vi "Vision Code.vi"(0 "Image In":T1, 1 "Image Dst":T1, 2 "Final Image Output":T1, 7 "error in":errorcluster) -> (20 "Image Out":T1, 22 "Output Image":T1(plugin-control), 27 "error out":errorcluster)   [LabVIEW 2014]
doc: "Creates, edits, and runs vision algorithms using NI Vision Assistant.\n\nWhen you place this Express VI on the block diagram, NI Vision Assistant launches. Create an algorithm using the Vision Assistant processing functions. After you create an algorithm, you can select the controls and indicators that you want to be able to programmatically set in LabVIEW. Double-click the Vision Assistant Express VI to edit the algorithm."
uses:
  <vilib>/vision/Image Controls.llb/IMAQ Image.ctl
  <vilib>/vision/NI_Vision_Development_Module.lvlib
panel:
  in  "Filter Parameters":T2={"Sigma"=1.0, "HThresh"=0.7, "LThres"=0.2, "WindowSize"=9} {"LThres" min=0 max=1 format="%.2f"; "HThresh" min=0 max=1 format="%.2f"; "Sigma" min=0 max=1 format="%.2f"}
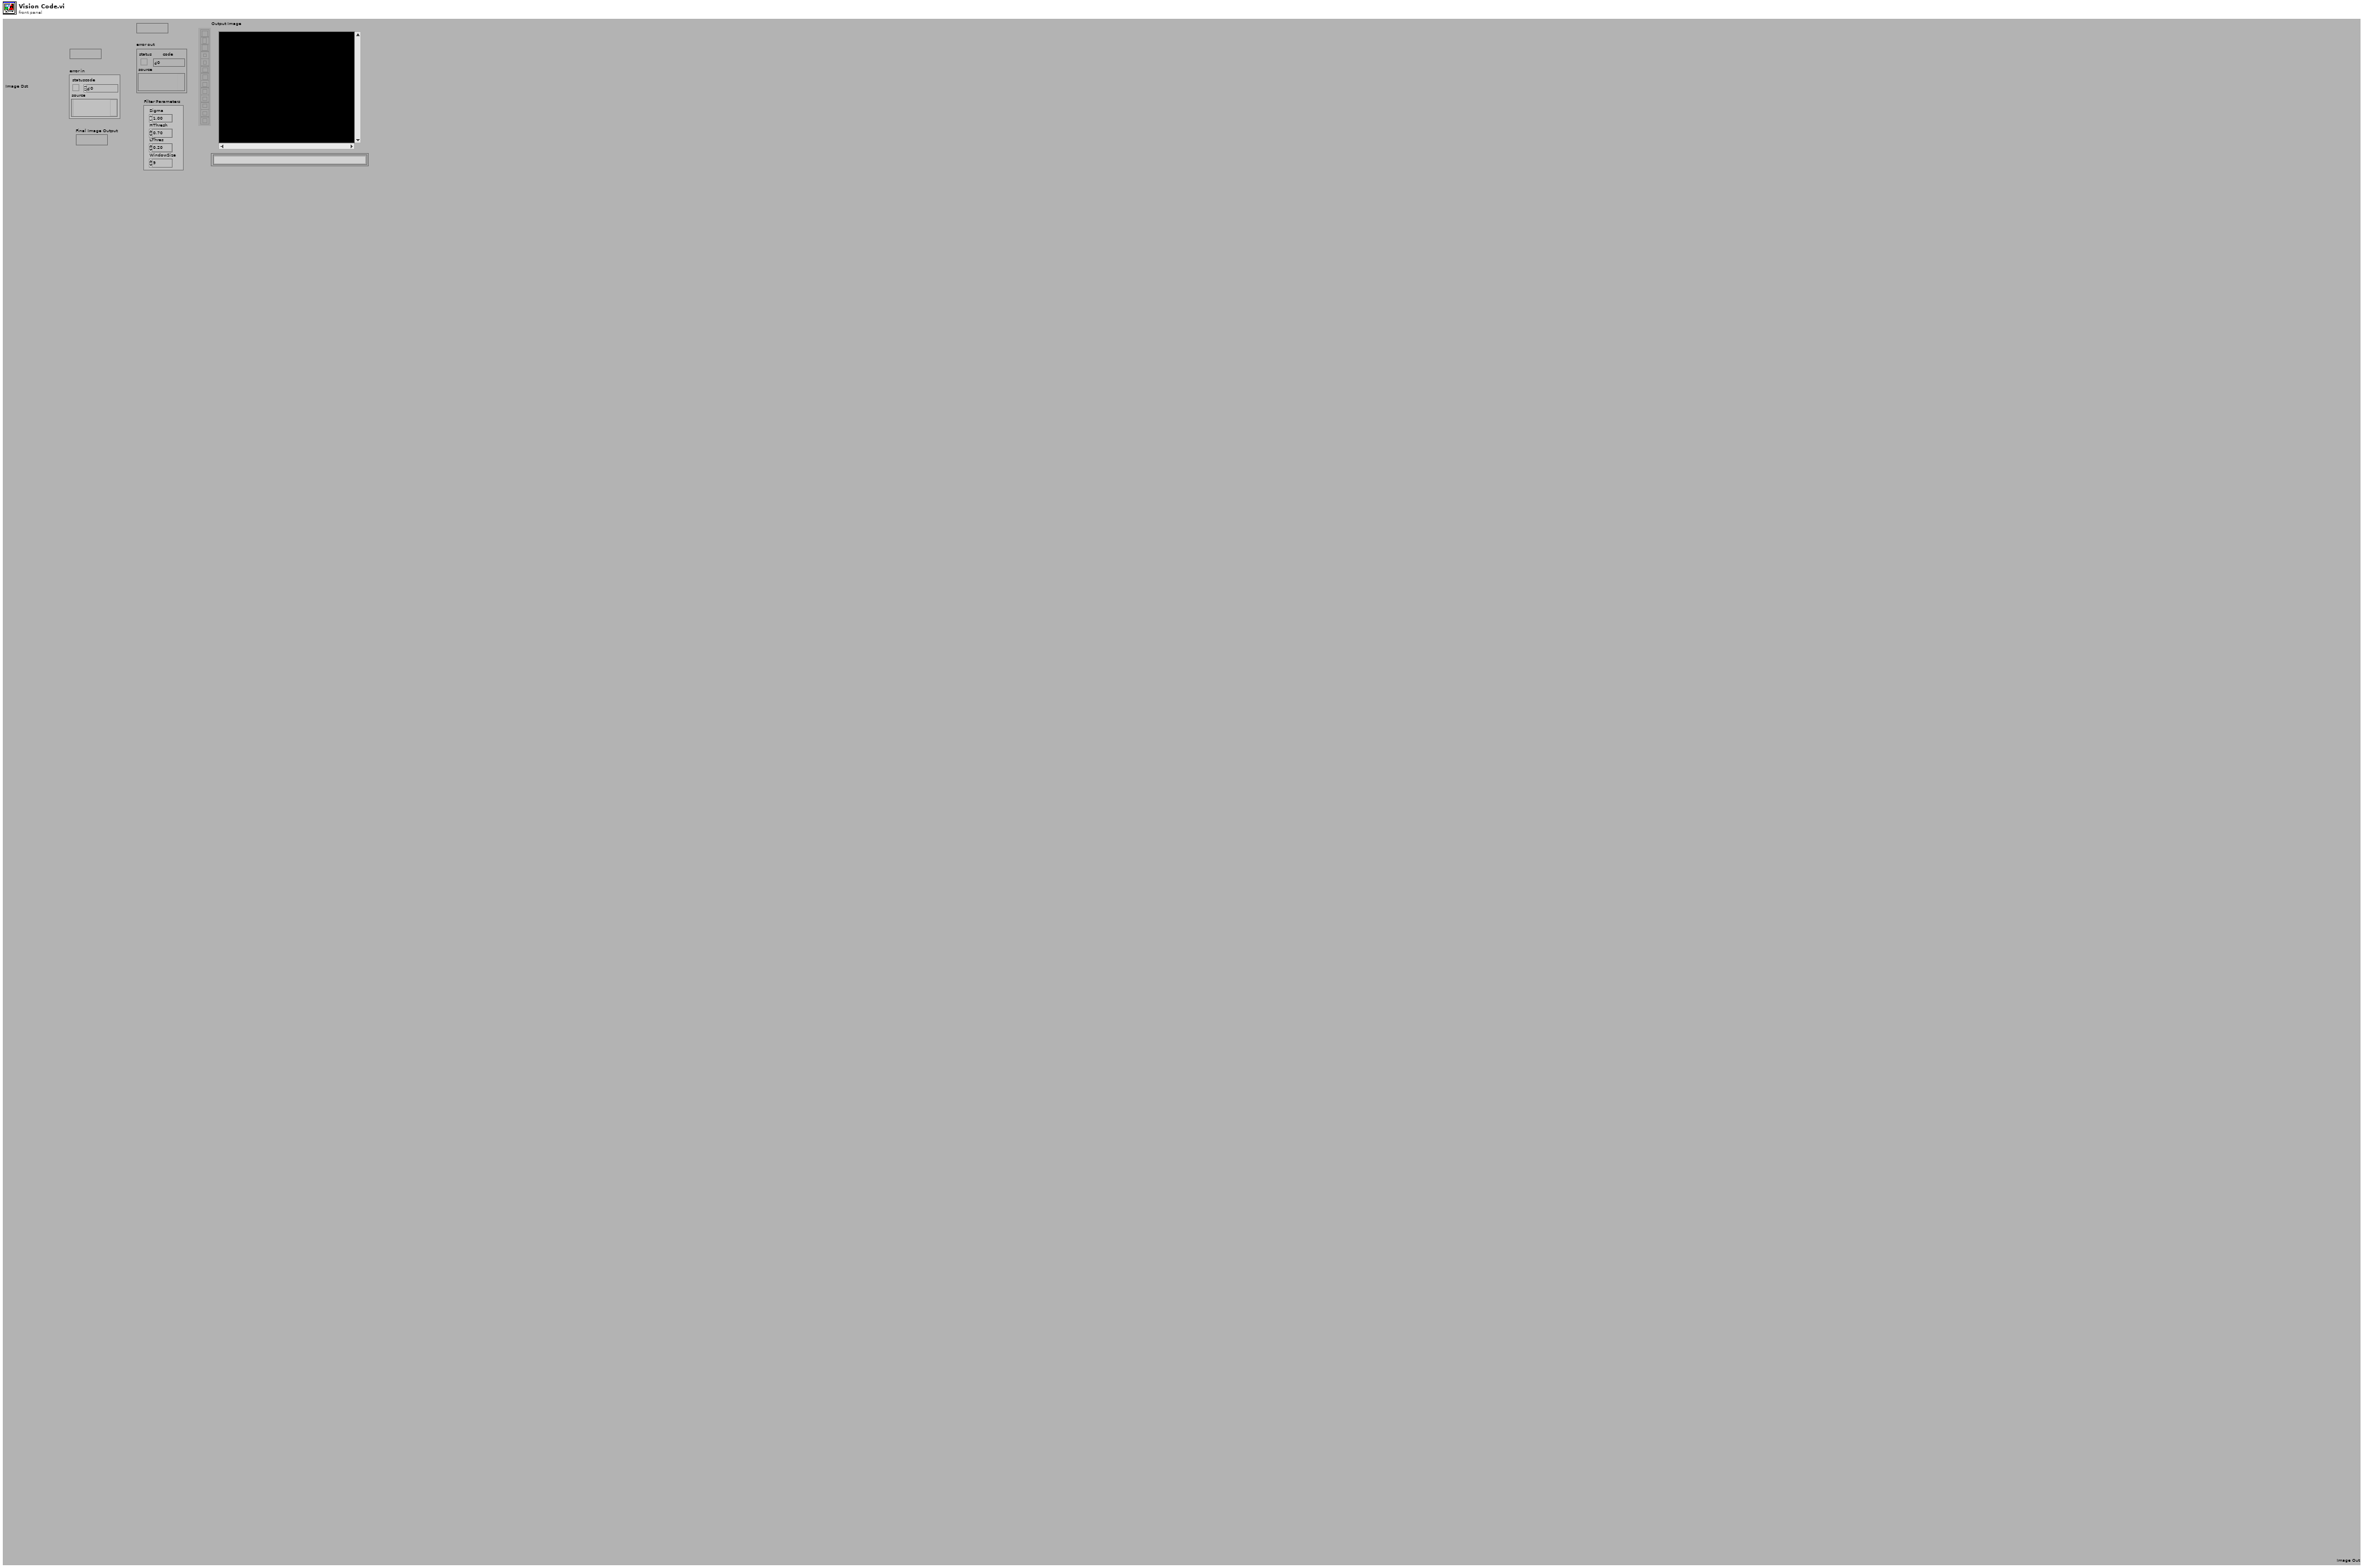
[diagram p1: front panel]
types:
  T1 = typedef "IMAQ Image.ctl" = refnum<image>
  T2 = cluster{"Sigma":sgl, "HThresh":sgl, "LThres":sgl, "WindowSize":i32}
  T3 = cluster{"Global Rectangle":i32[], "Contours":cluster{"ID":enum32{"External", "Internal"}, "Type":u32, "Coordinates":i32[]}[]}
  T4 = typedef "Image Type" = u32
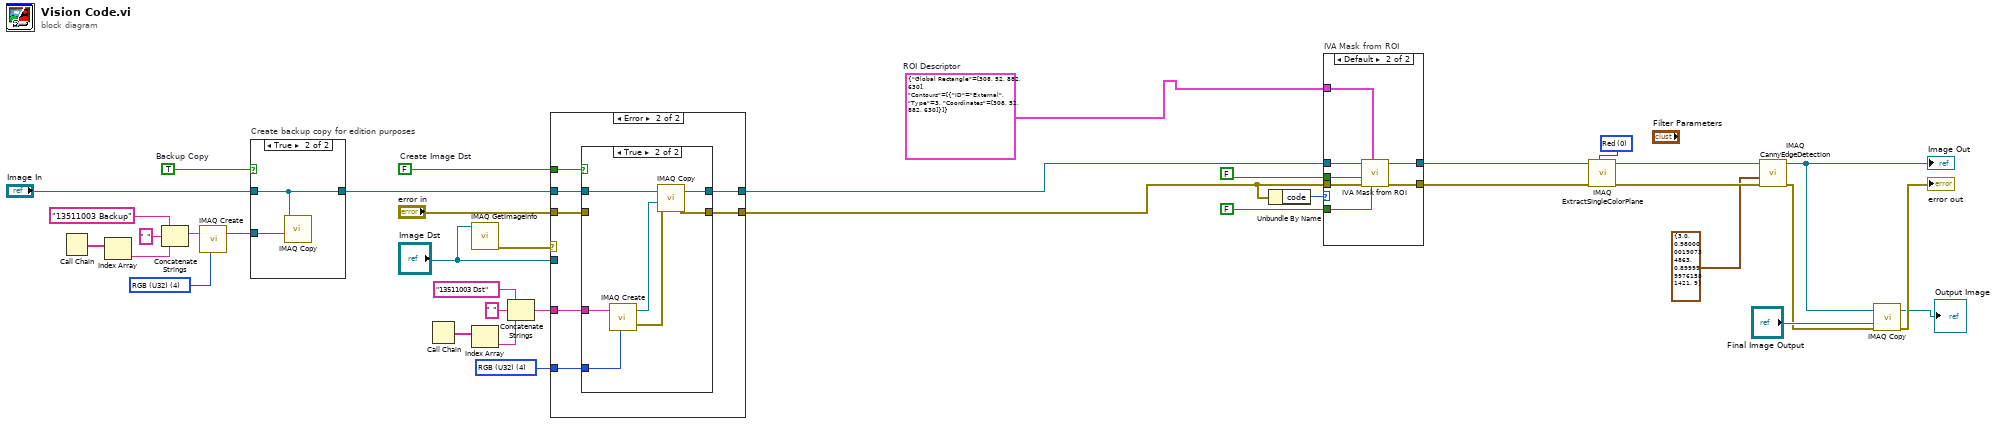
[diagram p0: block diagram]
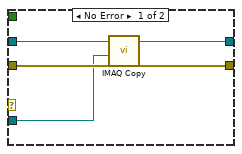
[diagram p3: hidden frame]
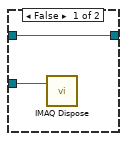
[diagram p5: hidden frame]
diagram:
  w10 = 0 items=["Red", "Green", "Blue", "Hue", "Saturation", "Luminance", "Value", "Intensity"] ("Color Plane")
  w16 = T3 {"Global Rectangle"=[308, 52, 882, 630], "Contours"=[{"ID"=enum."External", "Type"=3, "Coordinates"=[308, 52, 882, 630]}]}  # ROI Descriptor
  w17 = T4 4 items=["Grayscale (U8)", "Grayscale (I16)", "Grayscale (SGL)", "Complex (CSG)", "RGB (U32)", "HSL (U32)", "RGB (U64)", "Grayscale (U16)"] ("Image Dst Type")
  w18 = T4 4 items=["Grayscale (U8)", "Grayscale (I16)", "Grayscale (SGL)", "Complex (CSG)", "RGB (U32)", "HSL (U32)", "RGB (U64)", "Grayscale (U16)"] ("Image Type")
  w37 = TRUE  # Backup Copy
  w30 = FALSE  # Create Image Dst
  n1 = Call Chain() -> (call chain=w24:string[])
  n2 = Index Array(array=w24) -> (element=w23:string)  [unwired: 1 in]
  n3 = Concatenate Strings("13511003 Backup" ("Backup Image Name"), " ", w23) -> (w20:string)
  n4 = call "IMAQ Create"("Image Name"=w20, "Image Type"=w18) -> ("New Image"=w19:T1)  [unwired: 2 in, 2 out]
  n5 = case "Create backup copy for edition purposes" shown="True" w37 {
    tunnel: [w39 w41] -> w33
    tunnel: "Image In" -> [w39 w41]
    tunnel: w19 -> [w38 w40]
    frame False {
      n6 = call "IMAQ Dispose"("Image"=w38) -> ()  [unwired: 2 in, 4 out]
    }
    frame True {
      n7 = call "IMAQ Copy"("Image Dst"=w40, "Image Src"=w41) -> ()  [unwired: 1 in, 5 out]
    }
  }
  n8 = Call Chain() -> (call chain=w29:string[])
  n9 = call "IMAQ GetImageInfo"("Image"="Image Dst") -> ("error out"=w35:errorcluster)  [unwired: 1 in, 9 out]
  n10 = Index Array(array=w29) -> (element=w27:string)  [unwired: 1 in]
  n11 = Concatenate Strings("13511003 Dst" ("Image Dst Name"), " ", w27) -> (w25:string)
  n12 = case shown="Error" w35 {
    tunnel: [w46 w50] -> w14
    tunnel: [w45 w49] -> w31
    tunnel: w33 -> [w44 w51]
    tunnel: "error in" -> [w43 w47]
    tunnel: "Image Dst" -> [w42 _]
    tunnel: w25 -> [_ w53]
    tunnel: w17 -> [_ w52]
    tunnel: w30 -> [_ w48]
    frame No Error {
      n13 = call "IMAQ Copy"("error in (no error)"=w43, "Image Dst"=w42, "Image Src"=w44) -> ("error out"=w45:errorcluster, "Image Dst Out"=w46:T1)  [unwired: 3 out]
    }
    frame Error {
      n14 = case shown="True" w48 {
        tunnel: w53 -> [_ w62]
        tunnel: w52 -> [_ w61]
        tunnel: w51 -> [w55 w59]
        tunnel: [w55 w58] -> w50
        tunnel: [w54 w57] -> w49
        tunnel: w47 -> [w54 _]
        frame False {
        }
        frame True {
          n15 = call "IMAQ Create"("Image Name"=w62, "Image Type"=w61) -> ("New Image"=w60:T1, "error out"=w56:errorcluster)  [unwired: 2 in, 1 out]
          n16 = call "IMAQ Copy"("error in (no error)"=w56, "Image Dst"=w60, "Image Src"=w59) -> ("error out"=w57:errorcluster, "Image Dst Out"=w58:T1)  [unwired: 3 out]
        }
      }
    }
  }
  n17 = Unbundle By Name(w31) -> ("code"=w11:i32)
  n18 = case "IVA Mask from ROI" shown="Default" w11 {
    tunnel: w16 -> [_ w70]
    tunnel: FALSE ("Shrink") -> [_ w69]
    tunnel: w14 -> [w63 w68]
    tunnel: w31 -> [_ w67]
    tunnel: [_ w66] -> w13
    tunnel: [w63 w65] -> w9
    tunnel: FALSE ("Out / In") -> [_ w64]
    frame -1074396199, -1074396198 {
      # "Discard\nCoordinate\nSystem\nError"
    }
    frame Default {
      n19 = call <vilib>:"IVA Mask from ROI.vi"("Shrink"=w69, "ROI Descriptor"=w70, "error in (no error)"=w67, "Out / In"=w64, "Image Src"=w68) -> ("error out"=w66:errorcluster, "Image Out"=w65:T1)  [unwired: 5 out]
    }
  }
  n20 = call "IMAQ ExtractSingleColorPlane"("Color Plane"=w10, "error in (no error)"=w13, "Image Src"=w9) -> ("error out"=w8:errorcluster, "Image Dst Out"=w7:T1)  [unwired: 1 in, 6 out]
  n21 = call "IMAQ CannyEdgeDetection"("Image Src"=w7, "Filter Parameters"=T2 {"Sigma"=3.0, "HThresh"=0.98, "LThres"=0.9, "WindowSize"=9}, "error in (no error)"=w8) -> ("Image Dst Out"=w6:T1, "error out"=w4:errorcluster)  [unwired: 5 in]
  "Image Out" <- w6
  n22 = call "IMAQ Copy"("error in (no error)"=w4, "Image Dst"="Final Image Output", "Image Src"=w6) -> ("error out"=→"error out":errorcluster, "Image Dst Out"=→"Output Image":T1)  [unwired: 3 out]
